vi "pH_所有参数读取.vi"(8 "error in (no error)":errorcluster caption="错误输入（无错误）", 11 "MB session in":refnum<class "MB_Master.lvclass">) -> (0 "error out":errorcluster caption="错误输出", 2 "输出值":T1 {"电极型号标志" items=["NULL", "pH", "Cond", "DO", "Turb"]; "电极状态标志" items=["OK", "第一点校正通过", "第二点校正通过", "校正失败,电极零点超出范围", "校正失败,电极斜率超出范围", "第三点校正通过"]}, 3 "MB session out":refnum<class "MB_Master.lvclass">)   [LabVIEW 2016, in "斯坦道多参数.lvlib"]
uses:
  <vilib>/Plasmionique/MB Master/MB_Master/MB_Master.lvclass
  <vilib>/Plasmionique/MB Master/MB Master.lvlib
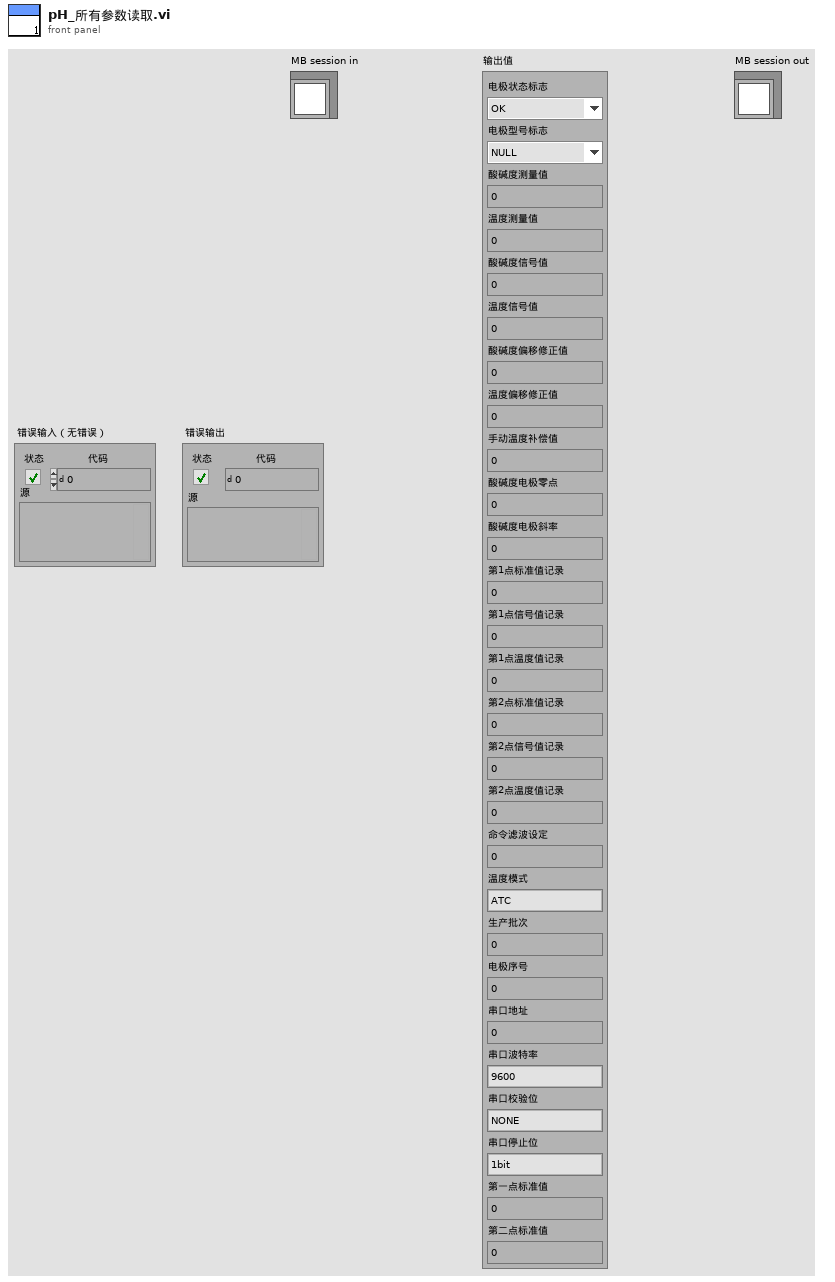
[diagram p1: front panel]
types:
  T1 = cluster{"电极状态标志":u16, "电极型号标志":u16, "酸碱度测量值":sgl, "温度测量值":sgl, "酸碱度信号值":sgl, "温度信号值":sgl, "酸碱度偏移修正值":sgl, "温度偏移修正值":sgl, "手动温度补偿值":sgl, "酸碱度电极零点":sgl, "酸碱度电极斜率":sgl, "第1点标准值记录":sgl, "第1点信号值记录":sgl, "第1点温度值记录":sgl, "第2点标准值记录":sgl, "第2点信号值记录":sgl, "第2点温度值记录":sgl, "命令滤波设定":u16, "温度模式":enum16{"ATC", "MTC"}, "生产批次":u16, "电极序号":u16, "串口地址":u16, "串口波特率":enum16{"9600", "19200", "115200"}, "串口校验位":enum16{"NONE", "ODD", "EVEN"}, "串口停止位":enum16{"1bit", "2bit"}, "第一点标准值":sgl, "第二点标准值":sgl}
  T2 = cluster{u16, u16, "数值":sgl, "数值":sgl, "数值":sgl, "数值":sgl, "数值":sgl, "数值":sgl, "数值":sgl, "数值":sgl, "数值":sgl, "数值":sgl, "数值":sgl, "数值":sgl, "数值":sgl, "数值":sgl, "数值":sgl, u16, u16, u16, u16, u16, u16, u16, u16, "数值":sgl, "数值":sgl}
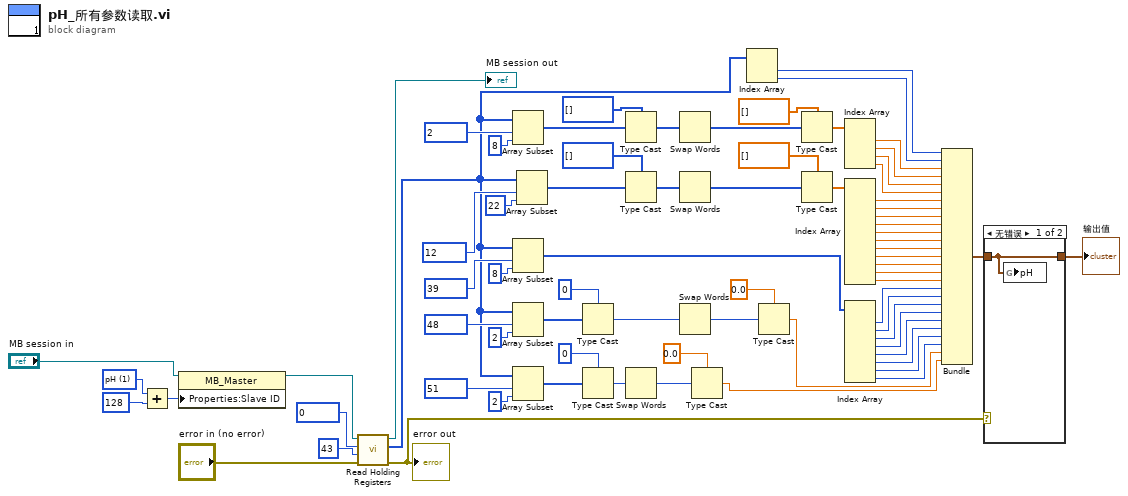
[diagram p0: block diagram]
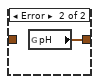
[diagram p2: hidden frame]
diagram:
  w73 = u16 1 items=["NULL", "pH", "Cond", "DO", "Turb"] ("数值")
  n1 = Add(x=w73, y=u16 128) -> (x+y=w72:u16)
  n2 = property class="MB_Master"(reference="MB session in", "Properties:Slave ID"=w72) -> (reference out=w7:refnum<class "MB_Master.lvclass">)  [unwired: 1 in, 1 out]
  n3 = call <vilib>:"Read Holding Registers.vi"("error in (no error)"="error in (no error)", "quantity"=u16 43, "starting address"=u16 0, "MB session in"=w7) -> ("error out"=w6:errorcluster, "Registers"=w21:u16[], "MB session out"=→"MB session out":refnum<class "MB_Master.lvclass">)  [unwired: 5 in]
  "error out" <- w6
  n4 = Array Subset(array=w21, index=u16 2 ("starting address"), length=8 ("长度")) -> (w61:u16[])
  n5 = Array Subset(array=w21, index=u16 39 ("starting address"), length=8 ("长度")) -> (w34:u16[])
  n6 = Array Subset(array=w21, index=u16 48 ("starting address"), length=2 ("长度")) -> (w16:u16[])
  n7 = Array Subset(array=w21, index=u16 51 ("starting address"), length=2 ("长度")) -> (w11:u16[])
  n8 = Array Subset(array=w21, index=u16 12 ("starting address"), length=22 ("长度")) -> (w51:u16[])
  n9 = Type Cast(type=u32 0 ("数值"), x=w16) -> (*(type *) &x=w19:u32)
  n10 = Type Cast(type=u32 0 ("数值"), x=w11) -> (*(type *) &x=w13:u32)
  n11 = Type Cast(type=u32[] [] ("数组 2"), x=w61) -> (*(type *) &x=w63:u32[])
  n12 = Type Cast(type=u32[] [] ("数组 2"), x=w51) -> (*(type *) &x=w54:u32[])
  n13 = Swap Words(1:w13) -> (0:w12:u32)
  n14 = Swap Words(1:w63) -> (0:w65:u32[])
  n15 = Swap Words(1:w54) -> (0:w55:u32[])
  n16 = Swap Words(1:w19) -> (0:w20:u32)
  n17 = Type Cast(type=sgl 0.0 ("数值"), x=w12) -> (*(type *) &x=w9:sgl)
  n18 = Index Array(array=w21) -> (element #1=w68:u16, element #2=w67:u16)  [unwired: 2 in]
  n19 = Type Cast(type=sgl 0.0 ("数值"), x=w20) -> (*(type *) &x=w10:sgl)
  n20 = Type Cast(type=sgl[] [] ("数组 2"), x=w65) -> (*(type *) &x=w60:sgl[])
  n21 = Type Cast(type=sgl[] [] ("数组 2"), x=w55) -> (*(type *) &x=w50:sgl[])
  n22 = Index Array(array=w60) -> (element #1=w2:sgl, element #2=w59:sgl, element #3=w58:sgl, element #4=w57:sgl)  [unwired: 4 in]
  n23 = Index Array(array=w50) -> (element #1=w49:sgl, element #2=w48:sgl, element #3=w47:sgl, element #4=w46:sgl, element #5=w45:sgl, element #6=w44:sgl, element #7=w43:sgl, element #8=w42:sgl, element #9=w41:sgl, element #10=w40:sgl, element #11=w39:sgl)  [unwired: 11 in]
  n24 = Index Array(array=w34) -> (element #1=w33:u16, element #2=w32:u16, element #3=w31:u16, element #4=w30:u16, element #5=w29:u16, element #6=w28:u16, element #7=w27:u16, element #8=w26:u16)  [unwired: 8 in]
  n25 = Bundle(w68, w67, "数值"=w2, "数值"=w59, "数值"=w58, "数值"=w57, "数值"=w49, "数值"=w48, "数值"=w47, "数值"=w46, "数值"=w45, "数值"=w44, "数值"=w43, "数值"=w42, "数值"=w41, "数值"=w40, "数值"=w39, w33, w32, w31, w30, w29, w28, w27, w26, "数值"=w10, "数值"=w9) -> (w5:T2)  [unwired: 1 in]
  n26 = case shown="无错误" w6 {
    tunnel: w5 -> [w74 _]
    tunnel: [w74 w75] -> w1
    frame No Error {
      n27 = global write "国弘过程全局变量.vi" "pH"(w74) -> ()
    }
    frame Error {
      n28 = global read "国弘过程全局变量.vi" "pH"() -> (w75:T1)
    }
  }
  "输出值" <- w1
